vi "SOUR_POW_COUP.vi"(0 "VISA IN":refnum<visa-resource-name>, 1 "Coupling ON/OFF":bool, 5 "error in":errorcluster, 7 "Channel":i32) -> (14 "VISA Out":refnum<visa-resource-name>, 19 "error out":errorcluster)   [LabVIEW 2018, in "PNA-X.lvlib"]
doc: "SOURce<cnum>:POWer:COUPle <ON | OFF> \n(Read-Write) Turns Port Power Coupling ON or OFF. \nParameters \n<cnum> Any existing channel number. If unspecified, value is set to 1 \n<ON | OFF> ON (or 1) - turns coupling ON. The same power level is used for both source \nports. \nOFF (or 0) - turns coupling OFF. Power level can be set individually for each \nsource port. \nExamples SOUR:POW:COUP ON \nsource2:power:couple off \nQuery Syntax SOURce<cnum>:POWer:COUPle? \nReturn Type Boolean (1 = ON, 0 = OFF) \nDefault ON"
uses:
  PNA-X.lvlib
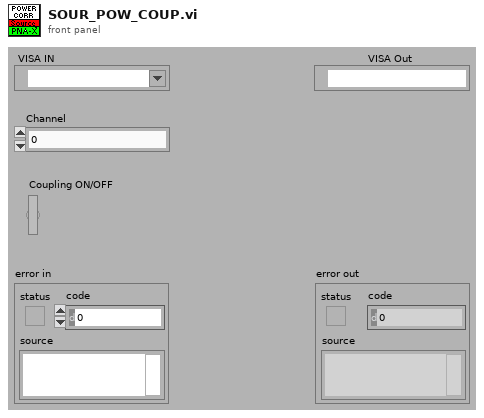
[diagram p1: front panel]
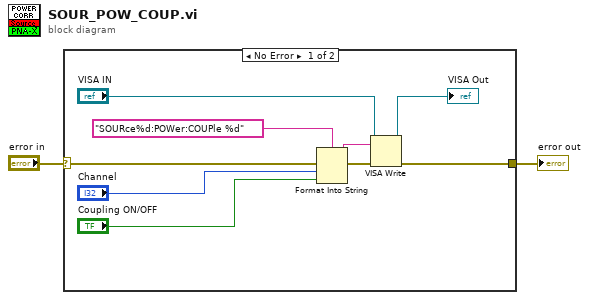
[diagram p0: block diagram]
diagram:
  n1 = case shown="No Error" "error in" {
    selector: "error in" -> [w11 w12]
    tunnel: [w6 w12] -> w1
    frame No Error {
      n2 = Format Into String(format string="SOURce%d:POWer:COUPle %d" ("Cmdline"), error in=w11, "Channel", "Coupling ON/OFF") -> (resulting string=w9:string, error out=w10:errorcluster)  [unwired: 1 in]
      n3 = VISA Write(VISA resource name="VISA IN", write buffer=w9, error in (no error)=w10) -> (VISA resource name out=→"VISA Out":refnum<visa-resource-name>, error out=w6:errorcluster)  [unwired: 1 out]
    }
    frame Error {
    }
  }
  "error out" <- w1
